vi "GetState_ClientID.vi"(8 "error in (no error)":errorcluster caption="错误输入（无错误）", 11 "TCPClientClass输入":refnum<class "TCPClientClass.lvclass">) -> (0 "error out":errorcluster caption="错误输出", 2 "连接ID":refnum<k5>, 3 "TCPClientClass输出":refnum<class "TCPClientClass.lvclass">)   [LabVIEW 2019, in "TCPClientClass.lvclass"]
uses:
  TCPClientClass.lvclass
  TCPClientClass.lvclass/TCPClientClass.ctl
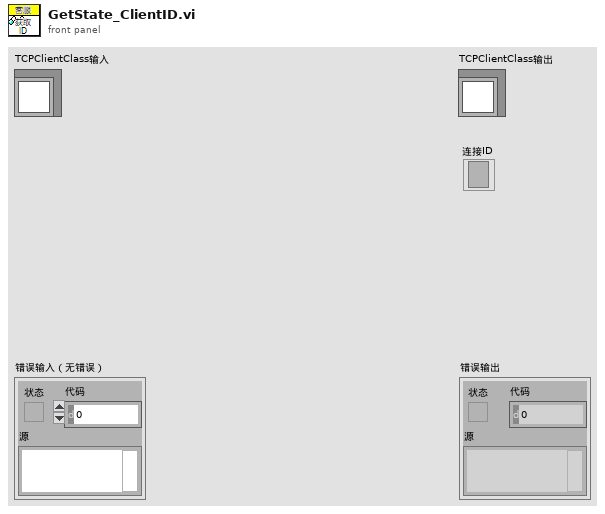
[diagram p1: front panel]
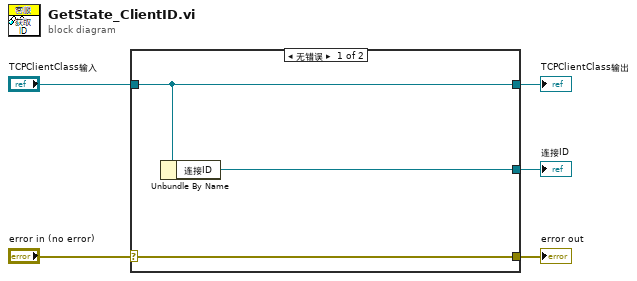
[diagram p0: block diagram]
diagram:
  n1 = case shown="无错误" "error in (no error)" {
    selector: "error in (no error)" -> [w8 w9]
    tunnel: [w8 w9] -> w4
    tunnel: [w7 w10] -> w2
    tunnel: "TCPClientClass输入" -> [w7 w10]
    tunnel: [w6 _] -> w1
    frame No Error {
      n2 = Unbundle By Name(w7) -> ("连接ID"=w6:refnum<k5>)
    }
    frame Error {
    }
  }
  "error out" <- w4
  "TCPClientClass输出" <- w2
  "连接ID" <- w1
